vi "get timing source.vi"(8 "error in":errorcluster, 11 "module configuration in":refnum<class "asynchronous execution module configuration.lvclass">) -> (0 "error out":errorcluster, 2 "timing source":T1, 3 "module configuration out":refnum<class "asynchronous execution module configuration.lvclass">)   [LabVIEW 2013, in "asynchronous execution module configuration.lvclass"]
doc: "An accessor which indicates whether or not the module is capable of generating a timing source for use with a timed loop or structure. This timing source can be enabled using <b>enable timing source.vi</b> and read using <b>read timing source.vi</b>."
uses:
  asynchronous execution module configuration.lvclass
  <vilib>/NI/Tag Bus Module Framework/module configuration/timing source.ctl
  asynchronous execution module configuration.lvclass/asynchronous execution module configuration.ctl
  <vilib>/NI/Tag Bus Module Framework/module configuration/TBM module configuration.lvclass
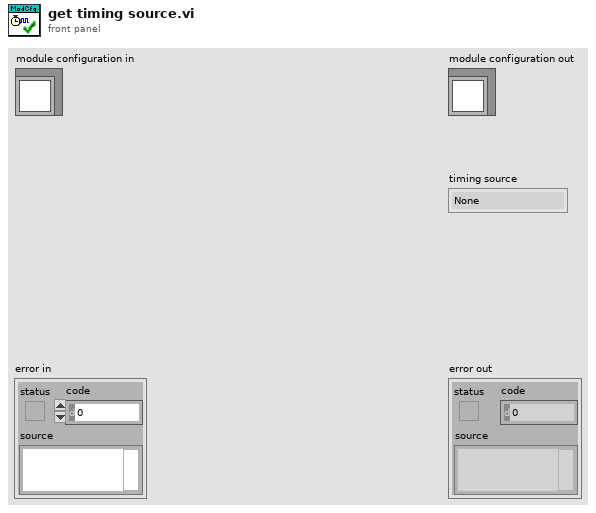
[diagram p1: front panel]
types:
  T1 = typedef "TBM module configuration.lvclass/timing source.ctl" = enum16{"None", "Custom Timing Source", "1 kHz Clock", "1 MHz Clock", "Synchronize to Scan Engine"}
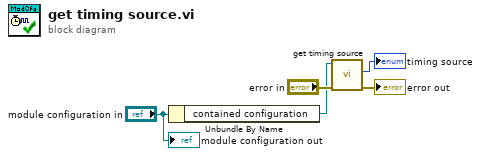
[diagram p0: block diagram]
diagram:
  n1 = Unbundle By Name("module configuration in") -> ("contained configuration"=w1:refnum<class "TBM module configuration.lvclass">)
  n2 = call-dynamic "get timing source.vi"("error in"="error in", "module configuration in"=w1) -> ("error out"=→"error out":errorcluster, "timing source enum"=→"timing source":T1)  [unwired: 7 in, 1 out]
  "module configuration out" <- "module configuration in"
